vi "Auton Builder.vi"() -> ()   [LabVIEW 2018]
uses:
  Typedef/Robot Settings.ctl
  Typedef/Data Point.ctl
  Typedef/Robot Starting Position.ctl
  Typedef/Sequence Command.ctl
  Typedef/Plate Arrangement.ctl
  <vilib>/Utility/miscctls.llb/LVRowAndColumnTypeDef.ctl
  <vilib>/Analysis/coordinate.llb/2D Cartesian Coordinate Rotation (Array).vi
  <vilib>/Analysis/coordinate.llb/2D Cartesian Coordinate Shift (Array).vi
  <vilib>/Analysis/NI_AALPro.lvlib
panel:
  in  "Start Position Names":T1
  in  "Stop?":bool
  in  "Tab Control":enum32{"Builder", "Raw Sequence", "Settings"}(tab)
  in  "Start Position":T1
  in  "Reverse Path":bool
  in  "Data Points":T2[](array[typedef])
  in  "Open":bool
  in  "Save":bool
  in  "Reset":bool
  in  "Send to Robot":bool
  in  "Simulate":bool
  in  "Name":string
  out "Field Half":cluster{dbl[], dbl[]}[](graph)
  in  "Cancel":bool
  out "Location Names":string[](array[string])
  in  "Locations":cluster{"X":dbl, "Y":dbl}[](array[cluster])=[{"X"=19.5, "Y"=162.0}, {"X"=0.0, "Y"=0.0}, {"X"=0.0, "Y"=0.0}, {"X"=0.0, "Y"=0.0}, {"X"=0.0, "Y"=0.0}]
  in  "Path Folder":path
  in  "Robot Settings":T3={"Width"=28.5, "Length"=33.5, "Center of Rotation"=19.5} caption="Robot Settings w/ Bumpers"
  # "LEFT"
  # "FAR"
  # "NEAR"
  # "RIGHT"
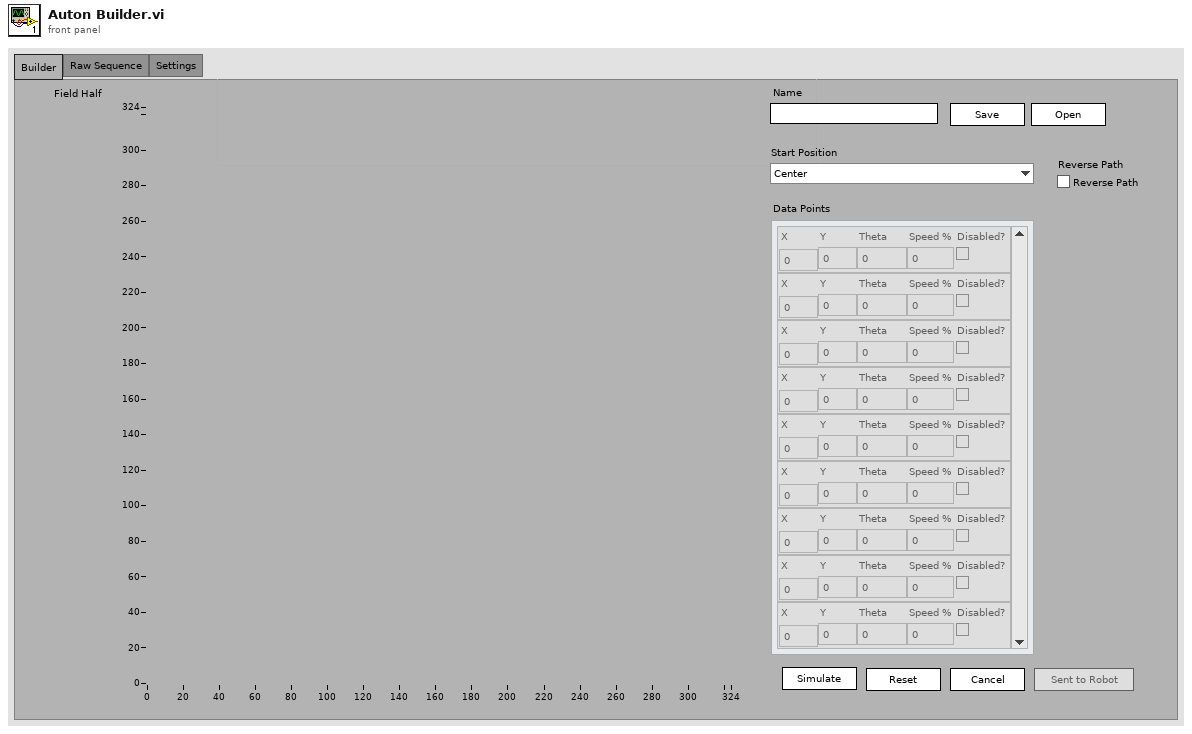
[diagram p1: front panel]
types:
  T1 = typedef "Robot Starting Position.ctl" = enum16{"Center", "Left Level 1", "Right Level 1", "Left Level 2", "Right Level 2"}
  T2 = typedef "Data Point.ctl" = cluster{"X":dbl, "Y":dbl, "Theta":dbl, "Speed %":dbl, "Disabled?":bool}
  T3 = typedef "Robot Settings.ctl" = cluster{"Width":dbl, "Length":dbl, "Center of Rotation":dbl}
  T4 = typedef "Sequence Command.ctl" = cluster{"Sequence Name":string, "Plate Arrangement":T5, "Command Name":string, "Data":variant, "Sequence Number":u32}
  T5 = typedef "Plate Arrangement.ctl" = cluster{"LR*":bool, "LL*":bool, "RL*":bool, "RR*":bool}
  T6 = typedef "LVRowAndColumnTypeDef.ctl" = cluster{"Row":i32, "Column":i32}
  T7 = cluster{"Field Half":cluster{dbl[], dbl[]}[], "Current Command":T4, "Robot Position":cluster{"x":dbl, "y":dbl}, "Theta":dbl, "y position":dbl, "Active Cell":T6, "Robot Index":i32, "Sequence OK?":bool, "Start Position":cluster{"x":dbl, "y":dbl}, "Field Selection":string, "Simulation Index":i32, "Sim Robot Index":i32, "Active Path":path, "Load Index":i32, "Graph Index":i32, "Data Points Index":i32, "Data Points":T2[], "Path Index":i32, "Path L Index":i32, "Path R Index":i32}
  T8 = typedef "LVPoint32TypeDef.ctl" = cluster{"Horizontal":i32, "Vertical":i32}
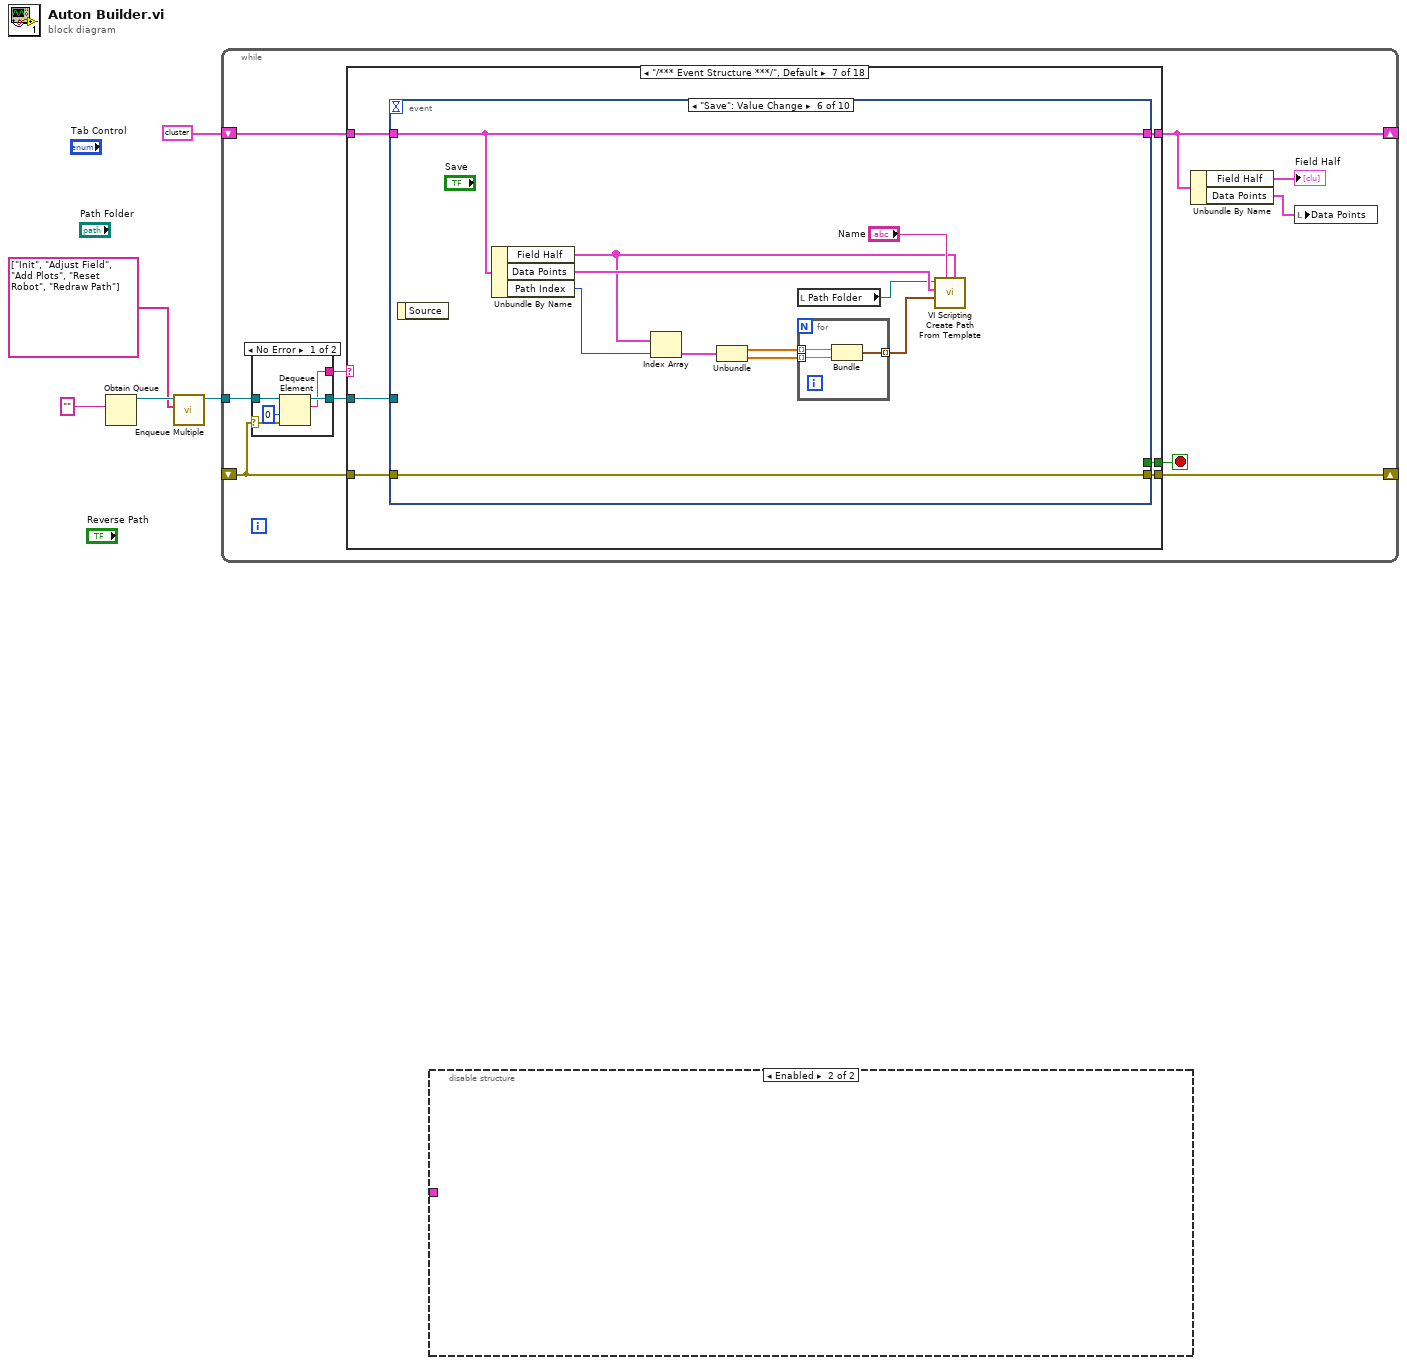
[diagram p0: block diagram]
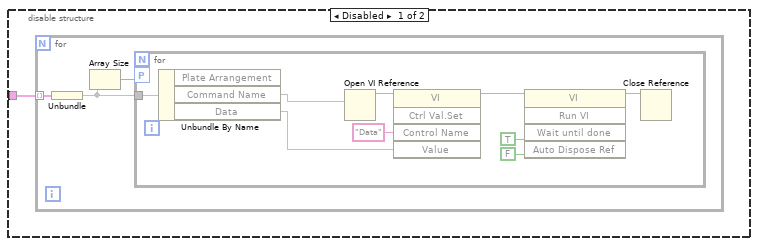
[diagram p2: hidden frame]
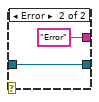
[diagram p3: hidden frame]
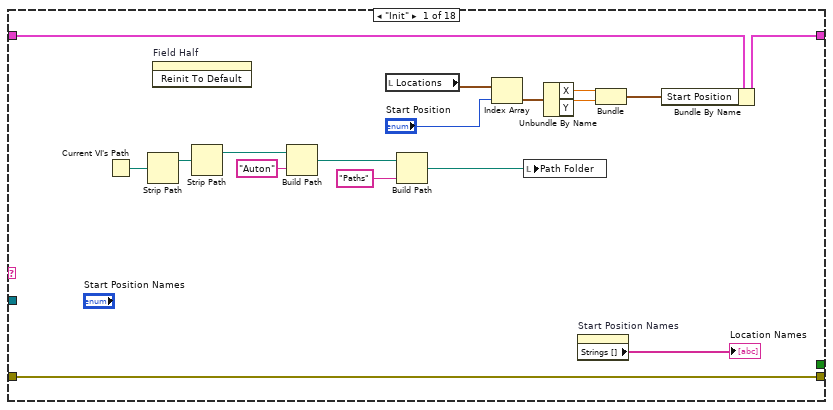
[diagram p4: hidden frame]
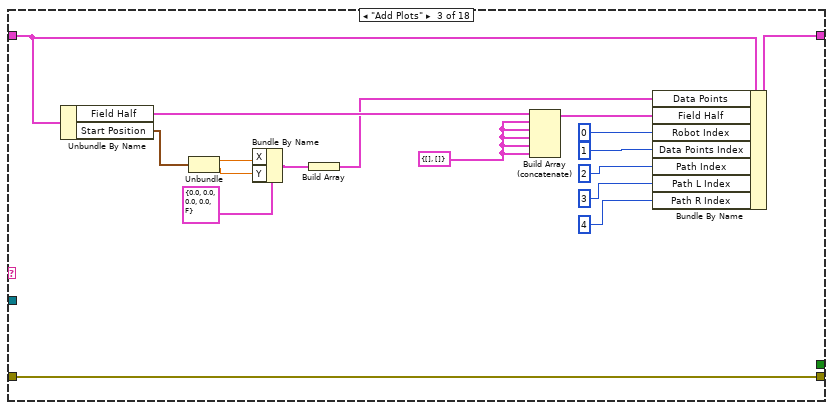
[diagram p6: hidden frame]
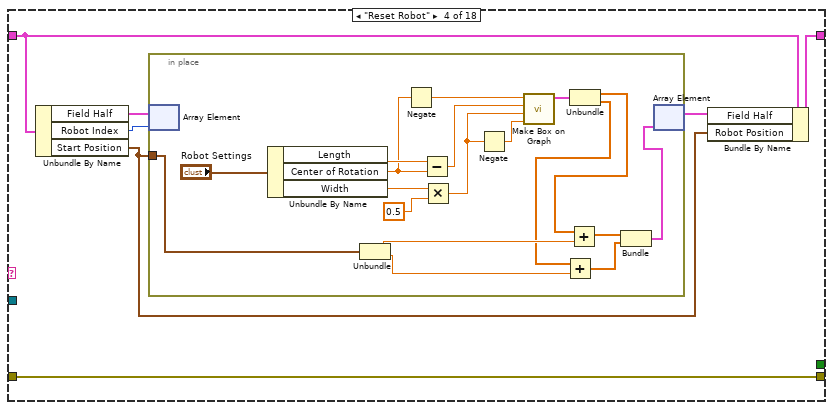
[diagram p7: hidden frame]
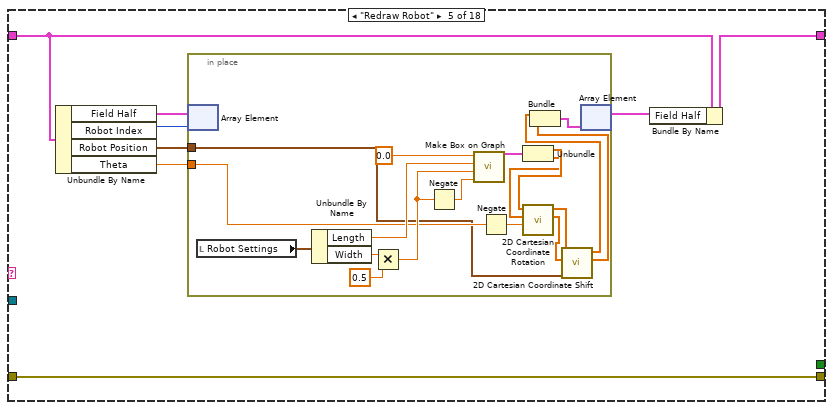
[diagram p8: hidden frame]
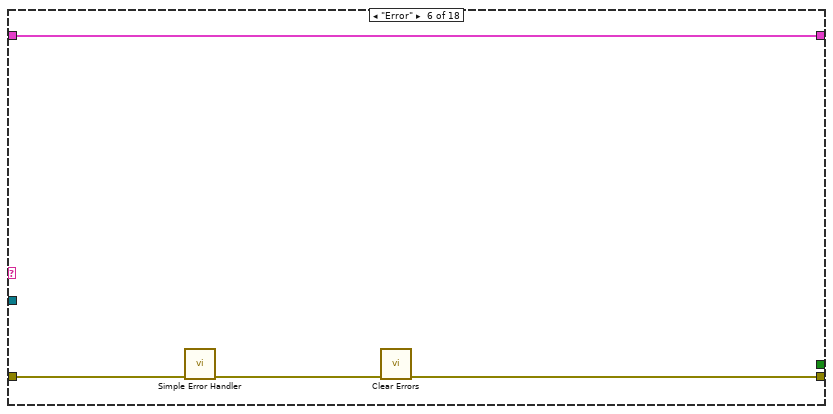
[diagram p9: hidden frame]
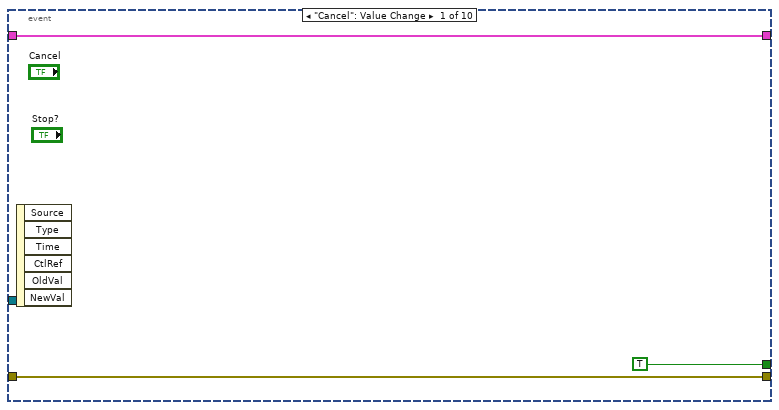
[diagram p10: hidden frame]
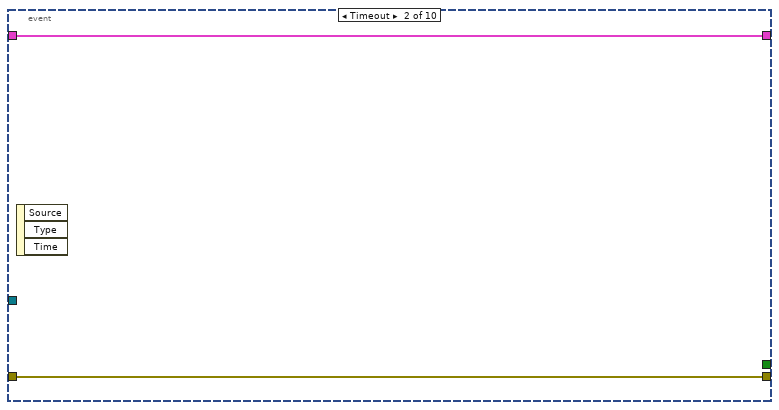
[diagram p11: hidden frame]
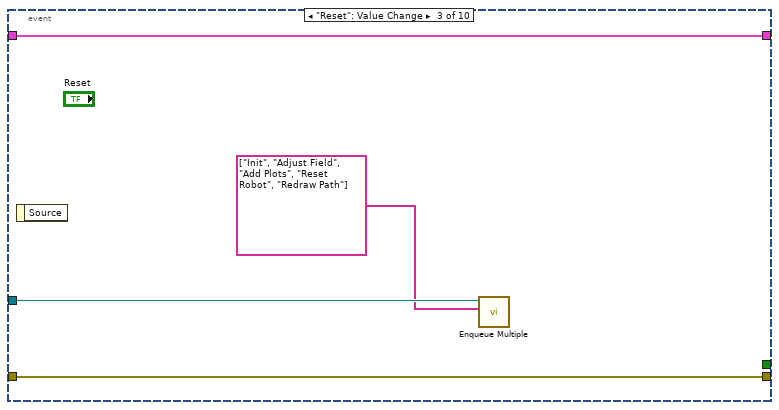
[diagram p12: hidden frame]
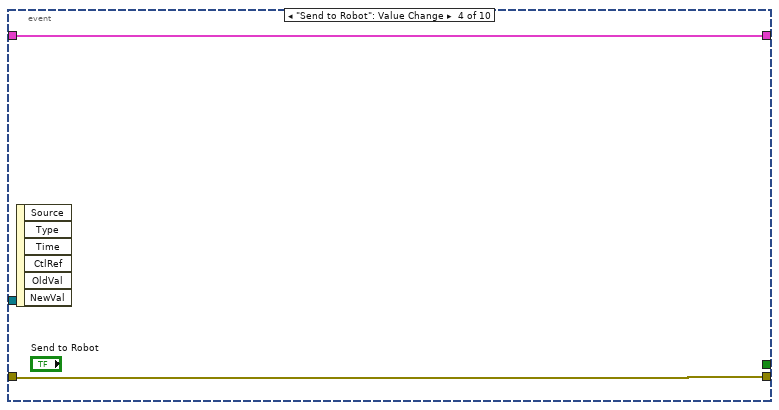
[diagram p13: hidden frame]
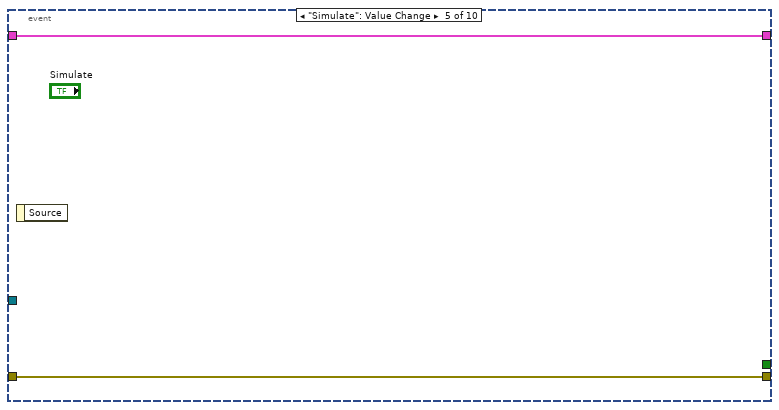
[diagram p14: hidden frame]
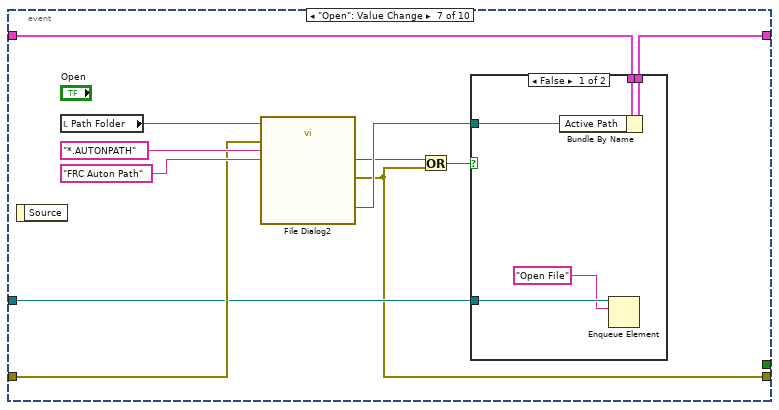
[diagram p15: hidden frame]
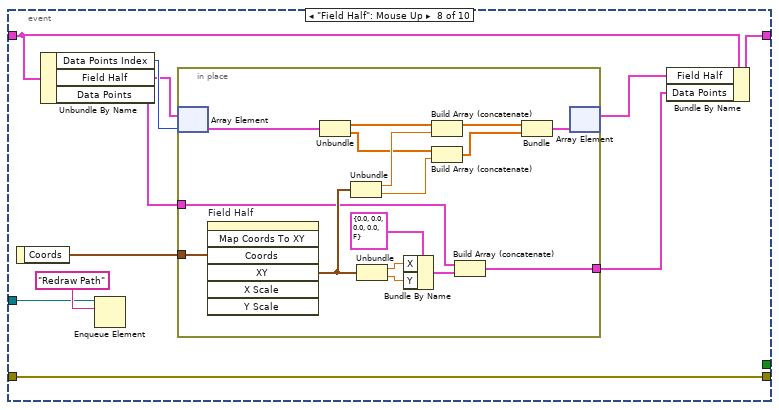
[diagram p17: hidden frame]
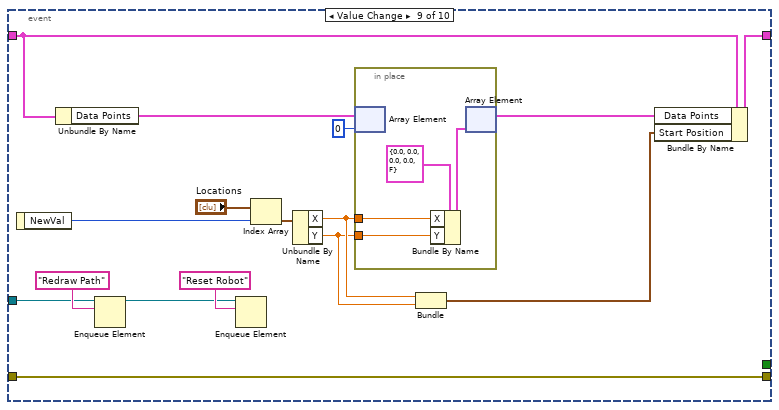
[diagram p18: hidden frame]
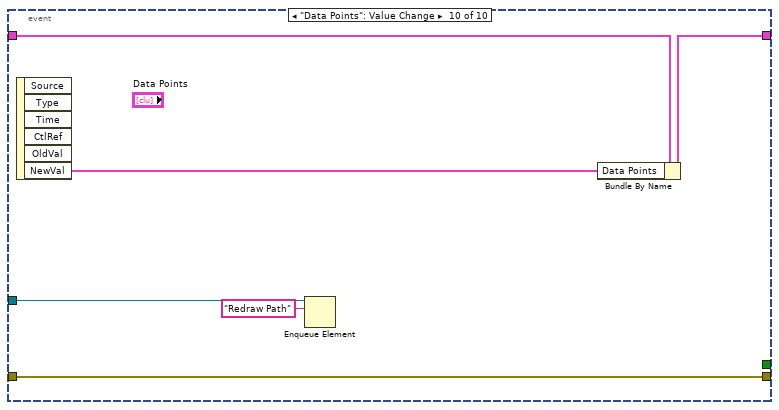
[diagram p19: hidden frame]
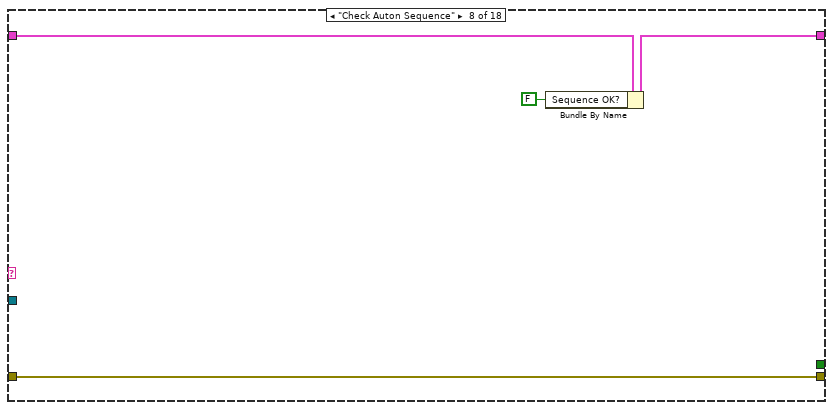
[diagram p20: hidden frame]
diagram:
  n1 = Obtain Queue(element data type="") -> (queue out=w4:refnum<queue>)  [unwired: 4 in, 2 out]
  n2 = call "Enqueue Multiple.vi"("Array"=string[] ["Init", "Adjust Field", "Add Plots", "Reset Robot", "Redraw Path"], "Queue in"=w4) -> ("Queue out"=w3:refnum<queue>)  [unwired: 8 in, 1 out]
  n3 = while {
    shift-right: [w9] -> _
    shift-left: T7 {"Field Half"=[], "Current Command"={"Sequence Name"="", "Plate Arrangement"={"LR*"=FALSE, "LL*"=FALSE, "RL*"=FALSE, "RR*"=FALSE}, "Command Name"="", "Data"=variant, "Sequence Number"=0}, "Robot Position"={"x"=0.0, "y"=0.0}, "Theta"=0.0, "y position"=0.0, "Active Cell"={"Row"=0, "Column"=0}, "Robot Index"=0, "Sequence OK?"=FALSE, "Start Position"={"x"=0.0, "y"=0.0}, "Field Selection"="", "Simulation Index"=0, "Sim Robot Index"=0, "Active Path"=path "", "Load Index"=0, "Graph Index"=0, "Data Points Index"=0, "Data Points"=[], "Path Index"=0, "Path L Index"=0, "Path R Index"=0} ("output cluster") -> [w15]
    shift-right: [w11] -> _
    shift-left: _ -> [w10]
    tunnel: w3 -> [w14]
    stop <- w7 stop-if-true
    n4 = case shown="No Error" w10 {
      selector: w10 -> [w18 _]
      tunnel: w14 -> [w20 w22]
      tunnel: [w19 w22] -> w13
      tunnel: [w17 "Error"] -> w12
      frame No Error {
        n5 = Dequeue Element(queue=w20, timeout in ms (-1)=0, error in (no error)=w18) -> (queue out=w19:refnum<queue>, element=w17:string)  [unwired: 2 out]
      }
      frame Error {
      }
    }
    n6 = case shown="\"/*** Event Structure ***/\", Default" w12 {
      tunnel: [_ _ _ _ _ _ w119 _ _ _ _ _ _ _ _ _ _ _] -> w7
      tunnel: w15 -> [w39 w40 w56 w64 w90 w113 w118 w219 w231 w246 w258 w272 w301 w306 w308 w310 w312 w314]
      tunnel: [w38 w40 w58 w65 w91 w113 w117 w218 w224 w242 w257 w270 w301 w304 w308 w310 w312 w314] -> w9
      tunnel: w13 -> [_ _ _ _ _ _ w116 _ _ _ _ _ _ _ _ _ _ _]
      tunnel: [w37 w41 w54 w63 w89 w112 w114 w220 w222 w240 w259 w273 w300 w305 w307 w309 w311 w313] -> w11
      tunnel: w10 -> [w37 w41 w54 w63 w89 w111 w115 w220 w222 w240 w259 w273 w300 w305 w307 w309 w311 w313]
      frame "Init" {
        n7 = Current VI's Path() -> (path=w36:path)
        n8 = Strip Path(path=w36) -> (stripped path=w35:path)  [unwired: 1 out]
        n9 = invoke on="Field Half" class="XYGraph (strict)" method="Reinit To Default"() -> ()  [unwired: 3 in, 3 out]
        n10 = Strip Path(path=w35) -> (stripped path=w34:path)  [unwired: 1 out]
        n11 = Build Path(base path=w34, name or relative path="Auton") -> (appended path=w32:path)
        n12 = local read "Locations"() -> (w24:cluster{"X":dbl, "Y":dbl}[])
        n13 = Build Path(base path=w32, name or relative path="Paths") -> (appended path=w30:path)
        n14 = Index Array(array=w24, index="Start Position") -> (element=w28:cluster{"X":dbl, "Y":dbl})
        n15 = local write "Path Folder"(w30) -> ()
        n16 = Unbundle By Name(w28) -> ("X"=w27:dbl, "Y"=w26:dbl)
        n17 = property on="Start Position Names" class="Enum (strict)"() -> ("Strings []"=→"Location Names":string[])  [unwired: 2 in, 2 out]
        n18 = Bundle("X"=w27, "Y"=w26) -> (w25:cluster{"X":dbl, "Y":dbl})  [unwired: 1 in]
        n19 = Bundle By Name(cluster=w39, "Start Position"=w25) -> (w38:T7)
      }
      frame "Adjust Field" {
      }
      frame "Add Plots" {
        w47 = cluster{dbl[], dbl[]} {[], []} ("element")
        n20 = Unbundle By Name(w56) -> ("Field Half"=w55:cluster{dbl[], dbl[]}[], "Start Position"=w48:cluster{"x":dbl, "y":dbl})
        n21 = Unbundle(w48) -> ("x"=w45:dbl, "y"=w44:dbl)
        n22 = Bundle By Name(cluster=T2 {"X"=0.0, "Y"=0.0, "Theta"=0.0, "Speed %"=0.0, "Disabled?"=FALSE} ("Cluster"), "X"=w45, "Y"=w44) -> (w43:T2)
        n23 = Build Array(w43) -> (w42:T2[])
        n24 = Build Array (concatenate)(w55, w47, w47, w47, w47, w47) -> (w57:cluster{dbl[], dbl[]}[])
        n25 = Bundle By Name(cluster=w56, "Data Points"=w42, "Field Half"=w57, "Robot Index"=0, "Data Points Index"=1 ("Spline Index"), "Path Index"=2 ("Spline Index"), "Path L Index"=3 ("Spline Index"), "Path R Index"=4 ("Spline Index")) -> (w58:T7)
      }
      frame "Reset Robot" {
        n26 = Unbundle By Name(w64) -> ("Field Half"=w62:cluster{dbl[], dbl[]}[], "Robot Index"=w61:i32, "Start Position"=w59:cluster{"x":dbl, "y":dbl})
        n27 = in-place {
          in-place-border: w59 -> [w83]
          n28 = in-place-array #1(w62, w61) -> ()  [unwired: 1 out]
          n29 = Unbundle By Name("Robot Settings") -> ("Length"=w73:dbl, "Center of Rotation"=w72:dbl, "Width"=w77:dbl)
          n30 = Unbundle(w83) -> ("x"=w82:dbl, "y"=w81:dbl)
          n31 = Negate(x=w72) -> (-x=w74:dbl)
          n32 = Subtract(x=w73, y=w72) -> (x-y=w71:dbl)
          n33 = Multiply(x=w77, y=0.5 ("x")) -> (x*y=w76:dbl)
          n34 = Negate(x=w76) -> (-x=w75:dbl)
          n35 = call "Make Box on Graph.vi"("Y2"=w75, "Y1"=w76, "X2"=w71, "X1"=w74) -> ("Output Graph"=w69:cluster{dbl[], dbl[]})  [unwired: 7 in]
          n36 = Unbundle(w69) -> (w68:dbl[], w67:dbl[])
          n37 = Add(x=w67, y=w81) -> (x+y=w80:dbl[])
          n38 = Add(x=w68, y=w82) -> (x+y=w79:dbl[])
          n39 = Bundle(w79, w80) -> (w66:cluster{dbl[], dbl[]})  [unwired: 1 in]
          n40 = in-place-array #1(w66) -> (w60:cluster{dbl[], dbl[]}[])  [unwired: 1 out]
        }
        n41 = Bundle By Name(cluster=w64, "Field Half"=w60, "Robot Position"=w59) -> (w65:T7)
      }
      frame "Redraw Robot" {
        n42 = Unbundle By Name(w90) -> ("Field Half"=w88:cluster{dbl[], dbl[]}[], "Robot Index"=w87:i32, "Robot Position"=w85:cluster{"x":dbl, "y":dbl}, "Theta"=w84:dbl)
        n43 = in-place {
          in-place-border: w85 -> [w96]
          in-place-border: w84 -> [w99]
          n44 = in-place-array #2(w88, w87) -> ()  [unwired: 1 out]
          n45 = local read "Robot Settings"() -> (w103:T3)
          n46 = Unbundle By Name(w103) -> ("Length"=w105:dbl, "Width"=w109:dbl)
          n47 = Multiply(x=w109, y=0.5 ("x")) -> (x*y=w107:dbl)
          n48 = Negate(x=w107) -> (-x=w106:dbl)
          n49 = call "Make Box on Graph.vi"("Y2"=w106, "Y1"=w107, "X2"=w105, "X1"=0.0) -> ("Output Graph"=w102:cluster{dbl[], dbl[]})  [unwired: 7 in]
          n50 = Negate(x=w99) -> (-x=w92:dbl)
          n51 = Unbundle(w102) -> (w101:dbl[], w100:dbl[])
          n52 = call-poly <vilib>:"2D Cartesian Coordinate Rotation.vi"("theta"=w92, "Y"=w100, "X"=w101) -> ("Y Out"=w97:dbl[], "X Out"=w98:dbl[])  [unwired: 6 in, 1 out]
          n53 = call-poly <vilib>:"2D Cartesian Coordinate Shift.vi"("shift"=w96, "Y"=w97, "X"=w98) -> ("Y Out"=w94:dbl[], "X Out"=w95:dbl[])  [unwired: 6 in, 1 out]
          n54 = Bundle("X Out"=w95, "Y Out"=w94) -> (w93:cluster{"X Out":dbl[], "Y Out":dbl[]})  [unwired: 1 in]
          n55 = in-place-array #2(w93) -> (w86:cluster{dbl[], dbl[]}[])  [unwired: 1 out]
        }
        n56 = Bundle By Name(cluster=w90, "Field Half"=w86) -> (w91:T7)
      }
      frame "Error" {
        n57 = call <vilib>:"Simple Error Handler.vi"("error in (no error)"=w111) -> ("error out"=w110:errorcluster)  [unwired: 4 in, 4 out]
        n58 = call <vilib>:"Clear Errors.vi"("error in (no error)"=w110) -> ("error out"=w112:errorcluster)  [unwired: 5 in, 1 out]
      }
      frame "/*** Event Structure ***/", Default {
        n59 = event shown="[5] \"Save\": Value Change" {
          selector: _ -> [_ _ _ _ _ _ _ _ _ _]
          dyn-events: _ -> [_ _ _ _ _ _ _ _ _ _]
          timeout: _ -> [_ _ _ _ _ _ _ _ _ _]
          tunnel: [TRUE _ _ _ _ _ _ _ _ _] -> w119
          tunnel: w118 -> [w121 w124 w128 w130 w132 w143 w151 w170 w205 w215]
          tunnel: [w121 w124 w128 w130 w132 w143 w150 w168 w204 w214] -> w117
          tunnel: w116 -> [_ _ w127 _ _ _ w153 w164 w202 w212]
          tunnel: w115 -> [w120 w123 w126 w129 w131 w139 w154 w174 w206 w216]
          tunnel: [w120 w123 w126 w129 w131 w139 w148 w174 w206 w216] -> w114
          event "Cancel": Value Change {
            n60 = event-data() -> ()  [unwired: 1 in, 6 out]
          }
          event Timeout {
            n61 = event-data() -> ()  [unwired: 1 in, 3 out]
          }
          event "Reset": Value Change {
            n62 = event-data() -> ()  [unwired: 1 in, 1 out]
            n63 = call "Enqueue Multiple.vi"("Array"=string[] ["Init", "Adjust Field", "Add Plots", "Reset Robot", "Redraw Path"], "Queue in"=w127) -> ()  [unwired: 8 in, 2 out]
          }
          event "Send to Robot": Value Change {
            n64 = event-data() -> ()  [unwired: 1 in, 6 out]
          }
          event "Simulate": Value Change {
            n65 = event-data() -> ()  [unwired: 1 in, 1 out]
          }
          event "Save": Value Change {
            n66 = event-data() -> ()  [unwired: 1 in, 1 out]
            n67 = Unbundle By Name(w143) -> ("Field Half"=w137:cluster{dbl[], dbl[]}[], "Data Points"=w141:T2[], "Path Index"=w136:i32)
            n68 = Index Array(array=w137, index=w136) -> (element=w135:cluster{dbl[], dbl[]})
            n69 = Unbundle(w135) -> (w133:dbl[], w134:dbl[])
            n70 = local read "Path Folder"() -> (w138:path)
            n71 = for {
              tunnel: [w146] -> w140 mode=indexing
              tunnel: w134 -> [w145] mode=indexing
              tunnel: w133 -> [w144] mode=indexing
              n72 = Bundle("x"=w144, "y"=w145) -> (w146:cluster{"x":dbl, "y":dbl})  [unwired: 1 in]
            }
            n73 = call "VI Scripting Create Path From Template.vi"("Graph"=w137, "Name"="Name", "path"=w140, "Data Points"=w141, "base path"=w138) -> ()  [unwired: 7 in]
          }
          event "Open": Value Change {
            n74 = event-data() -> ()  [unwired: 1 in, 1 out]
            n75 = local read "Path Folder"() -> (w157:path)
            n76 = call "File Dialog2"("start path"=w157, "error in"=w154, "pattern (all files)"="*.AUTONPATH", "pattern label"="FRC Auton Path") -> ("selected path"=w152:path, "cancelled"=w149:bool, "error out"=w148:errorcluster)  [unwired: 8 in, 1 out]
            n77 = Or(x=w149, y=w148) -> (x .or. y?=w147:bool)
            n78 = case shown="False" w147 {
              tunnel: w153 -> [w162 _]
              tunnel: w152 -> [w159 _]
              tunnel: w151 -> [w161 w163]
              tunnel: [w160 w163] -> w150
              frame False {
                n79 = Bundle By Name(cluster=w161, "Active Path"=w159) -> (w160:T7)
                n80 = Enqueue Element(queue=w162, element="Open File") -> ()  [unwired: 2 in, 3 out]
              }
              frame True {
              }
            }
          }
          event "Field Half": Mouse Up {
            n81 = event-data() -> ("Coords"=w173:T8)  [unwired: 1 in]
            n82 = Unbundle By Name(w170) -> ("Data Points Index"=w172:i32, "Field Half"=w171:cluster{dbl[], dbl[]}[], "Data Points"=w166:T2[])
            n83 = Enqueue Element(queue=w164, element="Redraw Path") -> ()  [unwired: 2 in, 3 out]
            n84 = in-place {
              in-place-border: w173 -> [w182]
              in-place-border: [w176] -> w167
              in-place-border: w166 -> [w175]
              n85 = in-place-array #3(w171, w172) -> (w190:cluster{dbl[], dbl[]})
              n86 = invoke on="Field Half" class="XYGraph (strict)" method="Map Coords To XY"("Coords"=w182) -> ("XY"=w180:cluster{"X":dbl, "Y":dbl})  [unwired: 6 in, 6 out]
              n87 = Unbundle(w190) -> (w188:dbl[], w187:dbl[])
              n88 = Unbundle(w180) -> ("X"=w189:dbl, "Y"=w186:dbl)
              n89 = Unbundle(w180) -> ("X"=w179:dbl, "Y"=w178:dbl)
              n90 = Bundle By Name(cluster=T2 {"X"=0.0, "Y"=0.0, "Theta"=0.0, "Speed %"=0.0, "Disabled?"=FALSE} ("Cluster"), "X"=w179, "Y"=w178) -> (w181:T2)
              n91 = Build Array (concatenate)(w188, w189) -> (w185:dbl[])
              n92 = Build Array (concatenate)(w187, w186) -> (w184:dbl[])
              n93 = Build Array (concatenate)(w175, w181) -> (w176:T2[])
              n94 = Bundle(w185, w184) -> (w183:cluster{dbl[], dbl[]})  [unwired: 1 in]
              n95 = in-place-array #3(w183) -> (w169:cluster{dbl[], dbl[]}[])  [unwired: 1 out]
            }
            n96 = Bundle By Name(cluster=w170, "Field Half"=w169, "Data Points"=w167) -> (w168:T7)
          }
          event Value Change {
            n97 = event-data() -> ("NewVal"=w196:T1)  [unwired: 1 in]
            n98 = Unbundle By Name(w205) -> ("Data Points"=w200:T2[])
            n99 = Enqueue Element(queue=w202, element="Redraw Path") -> (queue out=w194:refnum<queue>)  [unwired: 2 in, 2 out]
            n100 = Enqueue Element(queue=w194, element="Reset Robot") -> ()  [unwired: 2 in, 3 out]
            n101 = Index Array(array="Locations", index=w196) -> (element=w197:cluster{"X":dbl, "Y":dbl})
            n102 = Unbundle By Name(w197) -> ("X"=w193:dbl, "Y"=w192:dbl)
            n103 = in-place {
              in-place-border: w193 -> [w208]
              in-place-border: w192 -> [w207]
              n104 = in-place-array #4(w200, 0) -> ()  [unwired: 1 out]
              n105 = Bundle By Name(cluster=T2 {"X"=0.0, "Y"=0.0, "Theta"=0.0, "Speed %"=0.0, "Disabled?"=FALSE} ("element"), "X"=w208, "Y"=w207) -> (w210:T2)
              n106 = in-place-array #4(w210) -> (w201:T2[])  [unwired: 1 out]
            }
            n107 = Bundle("X"=w193, "Y"=w192) -> (w191:cluster{"X":dbl, "Y":dbl})  [unwired: 1 in]
            n108 = Bundle By Name(cluster=w205, "Data Points"=w201, "Start Position"=w191) -> (w204:T7)
          }
          event "Data Points": Value Change {
            n109 = event-data() -> ("NewVal"=w213:T2[])  [unwired: 1 in, 5 out]
            n110 = Enqueue Element(queue=w212, element="Redraw Path") -> ()  [unwired: 2 in, 3 out]
            n111 = Bundle By Name(cluster=w215, "Data Points"=w213) -> (w214:T7)
          }
        }
      }
      frame "Check Auton Sequence" {
        n112 = Bundle By Name(cluster=w219, "Sequence OK?"=FALSE) -> (w218:T7)
      }
      frame "Handle Graph Delete" {
        n113 = Unbundle By Name(w231) -> ("Field Half"=w225:cluster{dbl[], dbl[]}[], "Current Command"=w230:T4)
        n114 = Unbundle By Name(w230) -> ("Data"=w229:variant)
        n115 = Get Variant Attribute(Variant=w229, name="_graphIndex", default value (empty Variant)=0) -> (found=w221:bool, value=w227:i32)  [unwired: 1 in, 2 out]
        n116 = case shown="True" w221 {
          tunnel: w227 -> [_ w235]
          tunnel: w225 -> [w232 w234]
          tunnel: [w232 w233] -> w223
          frame False {
          }
          frame True {
            n117 = in-place {
              n118 = in-place-array #5(w234, w235) -> ()  [unwired: 1 out]
              n119 = in-place-array #5(cluster{dbl[], dbl[]} {[], []} ("element")) -> (w233:cluster{dbl[], dbl[]}[])  [unwired: 1 out]
            }
          }
        }
        n120 = Bundle By Name(cluster=w231, "Field Half"=w223) -> (w224:T7)
      }
      frame "Add Robot Plot" {
        n121 = Unbundle By Name(w246) -> ("Field Half"=w239:cluster{dbl[], dbl[]}[], "Current Command.Data"=w245:variant)
        n122 = Index Array(array=w239) -> (element=w237:cluster{dbl[], dbl[]})  [unwired: 1 in]
        n123 = Get Variant Attribute(Variant=w245, name="_graphPlot") -> (found=w243:bool, value=w238:variant)  [unwired: 2 in, 2 out]
        n124 = case shown="True" w243 {
          tunnel: [w247 w252] -> w241
          tunnel: w239 -> [w247 w251]
          tunnel: w238 -> [_ w250]
          tunnel: w237 -> [_ w249]
          frame False {
          }
          frame True {
            n125 = Variant To Data(type=w249, Variant=w250) -> (data=w248:cluster{dbl[], dbl[]})  [unwired: 1 in, 1 out]
            n126 = Build Array (concatenate)(w251, w248) -> (w252:cluster{dbl[], dbl[]}[])
          }
        }
        n127 = Bundle By Name(cluster=w246, "Field Half"=w241) -> (w242:T7)
      }
      frame "Update Graph Index" {
        n128 = Unbundle By Name(w258) -> ("Field Half"=w256:cluster{dbl[], dbl[]}[], "Graph Index"=w255:i32, "Current Command.Data"=w254:variant)
        n129 = in-place {
          in-place-border: w254 -> [w262]
          n130 = in-place-array #6(w256, w255) -> ()  [unwired: 1 out]
          n131 = Get Variant Attribute(Variant=w262, name="_graphPlot", default value (empty Variant)=cluster{dbl[], dbl[]} {[], []} ("value")) -> (value=w260:cluster{dbl[], dbl[]})  [unwired: 1 in, 3 out]
          n132 = in-place-array #6(w260) -> (w253:cluster{dbl[], dbl[]}[])  [unwired: 1 out]
        }
        n133 = Bundle By Name(cluster=w258, "Field Half"=w253) -> (w257:T7)
      }
      frame "Redraw Path" {
        n134 = Unbundle By Name(w272) -> ("Data Points"=w268:T2[], "Field Half"=w271:cluster{dbl[], dbl[]}[], "Data Points Index"=w264:i32, "Path Index"=w265:i32, "Path L Index"=w266:i32, "Path R Index"=w267:i32)
        n135 = in-place {
          in-place-border: w268 -> [w282]
          n136 = in-place-array #7(w271, w264, w265, w266, w267) -> ()  [unwired: 4 out]
          n137 = for {
            tunnel: [w299] -> w287 mode=indexing
            tunnel: w282 -> [w298] mode=indexing
            tunnel: [w297] -> w278 mode=indexing
            tunnel: [w296] -> w277 mode=indexing
            n138 = Unbundle(w298) -> ("X"=w297:dbl, "Y"=w296:dbl)  [unwired: 3 out]
            n139 = Bundle("X"=w297, "Y"=w296) -> (w299:cluster{"X":dbl, "Y":dbl})  [unwired: 1 in]
          }
          n140 = local read "Robot Settings"() -> (w275:T3)
          n141 = call "Path Inject Points.vi"("Distance"=1.0, "Path"=w287) -> ("Path out"=w292:cluster{dbl, dbl}[])  [unwired: 9 in]
          n142 = Bundle(w278, w277) -> (w276:cluster{dbl[], dbl[]})  [unwired: 1 in]
          n143 = Unbundle By Name(w275) -> ("Width"=w274:dbl)
          n144 = call "Path Smoother.vi"("tolerance"=0.001, "B"=0.95, "A"=0.05, "Path"=w292) -> ("SmoothPath"=w286:cluster{dbl, dbl}[])  [unwired: 7 in]
          n145 = for {
            tunnel: w286 -> [w295] mode=indexing
            tunnel: [w294] -> w284 mode=indexing
            tunnel: [w293] -> w285 mode=indexing
            n146 = Unbundle(w295) -> (w294:dbl, w293:dbl)
          }
          n147 = Bundle(w284, w285) -> (w279:cluster{dbl[], dbl[]})  [unwired: 1 in]
          n148 = call "Path to Wheel Path.vi"("Wheelbase (in)"=w274, "waypoints"=w279) -> ("out"=w283:cluster{dbl[], dbl[]}[])  [unwired: 9 in]
          n149 = Index Array(array=w283) -> (element #1=w280:cluster{dbl[], dbl[]}, element #2=w281:cluster{dbl[], dbl[]})  [unwired: 2 in]
          n150 = in-place-array #7(w276, w279, w280, w281) -> (w269:cluster{dbl[], dbl[]}[])  [unwired: 4 out]
        }
        n151 = Bundle By Name(cluster=w272, "Field Half"=w269) -> (w270:T7)
      }
      frame "/**** Simulation Functions ****/" {
      }
      frame "Simulation Init" {
        n152 = Bundle By Name(cluster=w306, "Simulation Index"=0, "Sim Robot Index"=0) -> (w304:T7)
      }
      frame "Select Field String" {
      }
      frame "/**** File Operations ****/" {
      }
      frame "Save File" {
      }
      frame "Open File" {
      }
    }
    n153 = Unbundle By Name(w9) -> ("Field Half"=→"Field Half":cluster{dbl[], dbl[]}[], "Data Points"=w6:T2[])
    n154 = local write "Data Points"(w6) -> ()
  }
  n155 = disable-structure shown="Enabled" {
    disable-tunnel: _ -> [w315 _]
    frame Disabled {
      n156 = for {
        tunnel: w315 -> [w318] mode=indexing
        n157 = Unbundle(w318) -> ("Sequence Array"=w316)
        n158 = Array Size(array=w316) -> (size(s)=w317:i32)
        n159 = for {
          tunnel: w316 -> [w327]
          workers-P: w317 -> [_]
          n160 = Unbundle By Name(w327) -> ("Command Name"=w323, "Data"=w325)  [unwired: 1 out]
          n161 = Open VI Reference(vi path=w323) -> (vi reference=w326:refnum<vi>)  [unwired: 5 in, 1 out]
          n162 = invoke class="VI" method="Ctrl Val.Set"(reference=w326, "Control Name"="Data", "Value"=w325) -> (reference out=w322:refnum<vi>)  [unwired: 2 in, 4 out]
          n163 = invoke class="VI" method="Run VI"(reference=w322, "Wait until done"=TRUE ("Wait Until Done"), "Auto Dispose Ref"=FALSE ("Auto Dispose Reference")) -> (reference out=w321:refnum<vi>)  [unwired: 2 in, 4 out]
          n164 = Close Reference(reference=w321) -> ()  [unwired: 1 in, 1 out]
        }
      }
    }
    frame Enabled {
    }
  }
